vi "Start Arrival Time Acquisition Temp File.vi"(8 "error in (no error)":errorcluster, 11 "Column Definitions":T2(array[cluster]) {"Offset" format="%.2f"; "Resolution" format="%.2f"}) -> (0 "error out":errorcluster, 3 "Temp File Definition":T1)   [LabVIEW 2009]
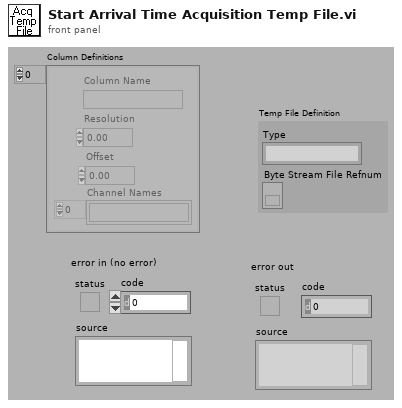
[diagram p1: front panel]
types:
  T1 = cluster{"Type":string, "Byte Stream File Refnum":refnum<file>}
  T2 = cluster{"Column Name":string, "Resolution":dbl, "Offset":dbl, "Channel Names":string[]}[]
  T3 = cluster{"Type":string, "refnum out":refnum<file>}
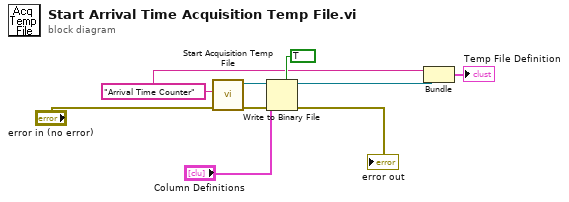
[diagram p0: block diagram]
diagram:
  w3 = "Arrival Time Counter" ("Type")
  n1 = call "Start Acquisition Temp File.vi"("error in (no error)"="error in (no error)", "Type"=w3) -> ("error out"=w7:errorcluster, "Byte Stream File Refnum"=w8:refnum<file>)  [unwired: 8 in]
  n2 = Write to Binary File(file (use dialog)=w8, data="Column Definitions", error in=w7, 5:TRUE ("header (F)")) -> (refnum out=w2:refnum<file>, error out=→"error out":errorcluster)  [unwired: 2 in, 1 out]
  n3 = Bundle("Type"=w3, "refnum out"=w2) -> (→"Temp File Definition":T3)  [unwired: 1 in]
